vi "message.vi"(5 "visible?":bool=TRUE, 8 "error in (no error)":errorcluster, 9 "BG slider":u32(colorbox)=16711680, 10 "text":string, 11 "control references in":T1) -> (0 "error out":errorcluster, 2 "previous text":string, 3 "control references out":T1, 4 "previously visible?":bool=TRUE, 6 "previous BG colour":u32(colorbox)=16711680)   [LabVIEW 2010]
uses:
  type_definitions/clusters/controls_refs.ctl
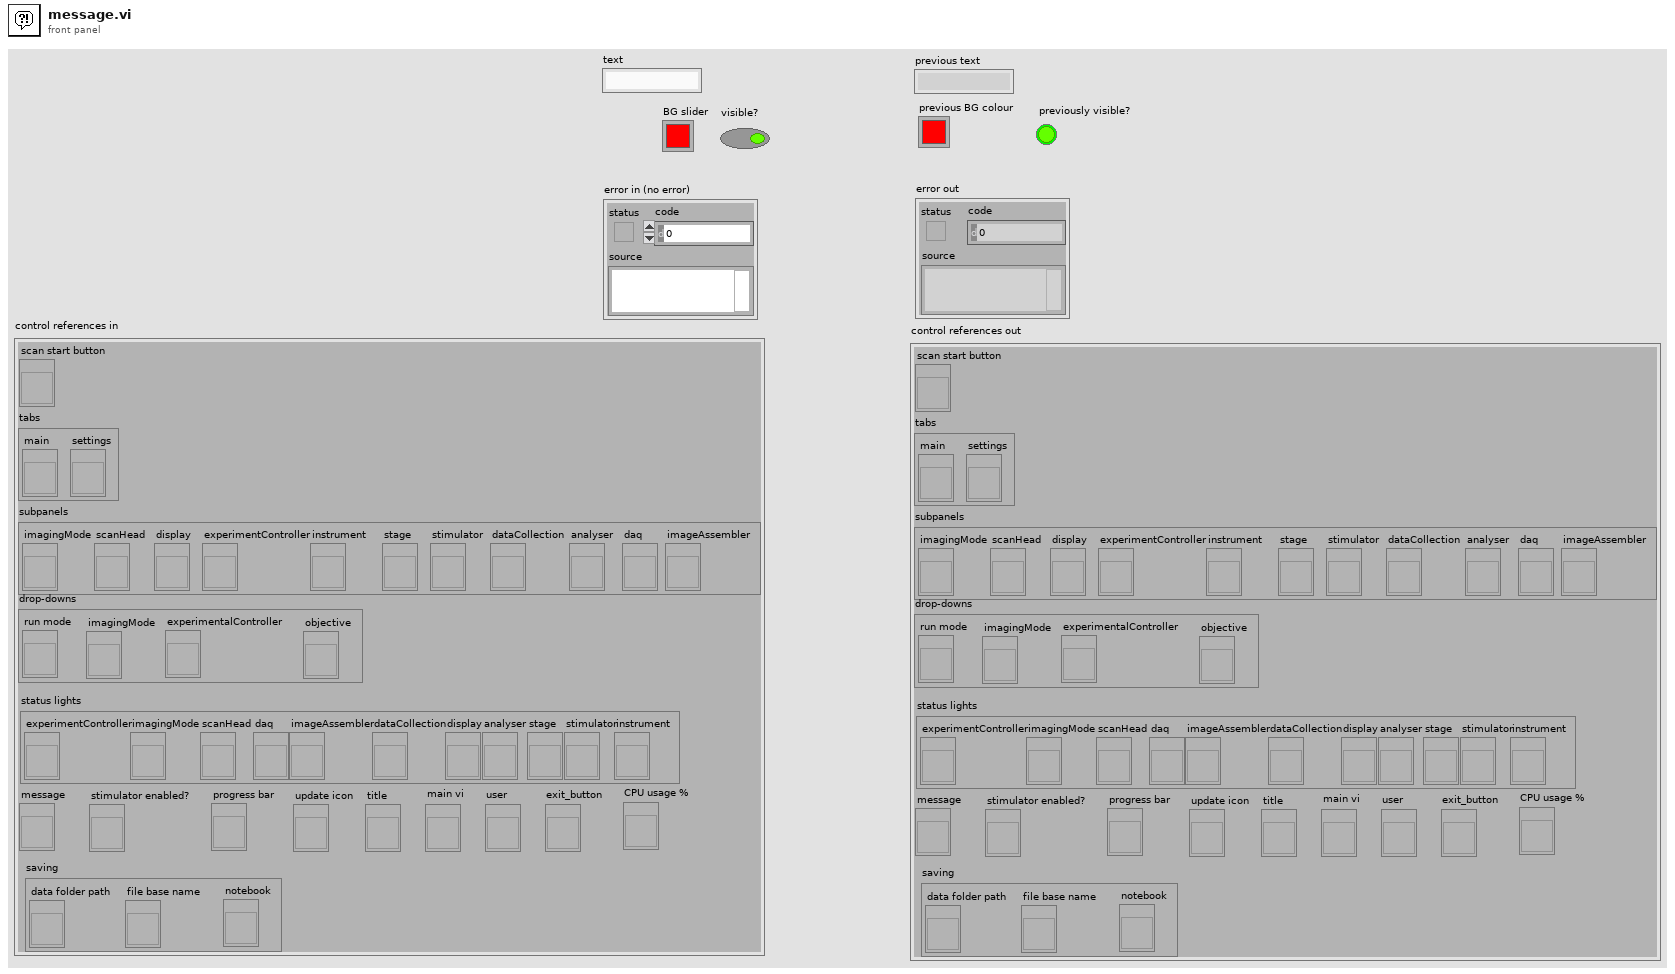
[diagram p1: front panel]
types:
  T1 = typedef "controls_refs.ctl" = cluster{"scan start button":refnum<vi>, "tabs":cluster{"main":refnum<vi>, "settings":refnum<vi>}, "subpanels":cluster{"imagingMode":refnum<vi>, "scanHead":refnum<vi>, "display":refnum<vi>, "experimentController":refnum<vi>, "instrument":refnum<vi>, "stage":refnum<vi>, "stimulator":refnum<vi>, "dataCollection":refnum<vi>, "analyser":refnum<vi>, "daq":refnum<vi>, "imageAssembler":refnum<vi>}, "drop-downs":cluster{"run mode":refnum<vi>, "imagingMode":refnum<vi>, "experimentalController":refnum<vi>, "objective":refnum<vi>}, "status lights":cluster{"experimentController":refnum<vi>, "imagingMode":refnum<vi>, "scanHead":refnum<vi>, "daq":refnum<vi>, "imageAssembler":refnum<vi>, "dataCollection":refnum<vi>, "display":refnum<vi>, "analyser":refnum<vi>, "stage":refnum<vi>, "stimulator":refnum<vi>, "instrument":refnum<vi>}, "message":refnum<vi>, "stimulator enabled?":refnum<vi>, "saving":cluster{"data folder path":refnum<vi>, "file base name":refnum<vi>, "notebook":refnum<vi>}, "progress bar":refnum<vi>, "update icon":refnum<vi>, "title":refnum<vi>, "main vi":refnum<vi>, "user":refnum<vi>, "exit_button":refnum<vi>, "CPU usage %":refnum<vi>}
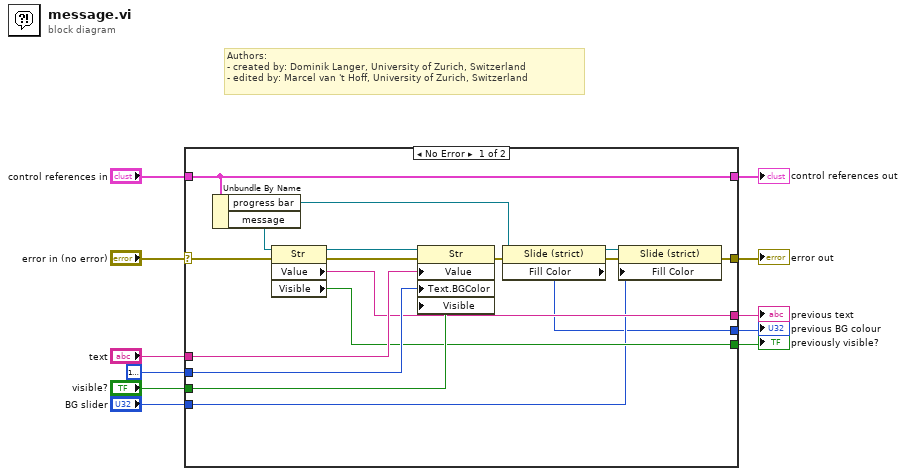
[diagram p0: block diagram]
diagram:
  # "Authors: \n- created by: Dominik Langer, University of Zurich, Switzerland\n- edited by: Marcel van 't Hoff, University of Zurich, Switzerland"
  n1 = case shown="No Error" "error in (no error)" {
    selector: "error in (no error)" -> [w21 w30]
    tunnel: [w18 w30] -> w10
    tunnel: "text" -> [w28 _]
    tunnel: u32 16777216 ("BG colour") -> [w27 _]
    tunnel: "visible?" -> [w26 _]
    tunnel: [w23 _] -> w5
    tunnel: [w12 _] -> w6
    tunnel: [w22 _] -> w4
    tunnel: "control references in" -> [w19 w29]
    tunnel: [w19 w29] -> w1
    tunnel: "BG slider" -> [w17 _]
    frame No Error {
      n2 = Unbundle By Name(w19) -> ("progress bar"=w14:refnum<vi>, "message"=w20:refnum<vi>)
      n3 = property class="Str"(reference=w20, error in=w21) -> (reference out=w24:refnum<vi>, error out=w25:errorcluster, "Value"=w23:string, "Visible"=w22:bool)
      n4 = property class="Str"(reference=w24, error in=w25, "Value"=w28, "Text.BGColor"=w27, "Visible"=w26) -> (error out=w16:errorcluster)  [unwired: 1 out]
      n5 = property class="Slide (strict)"(reference=w14, error in=w16) -> (reference out=w13:refnum<vi>, error out=w15:errorcluster, "Fill Color"=w12:u32)
      n6 = property class="Slide (strict)"(reference=w13, error in=w15, "Fill Color"=w17) -> (error out=w18:errorcluster)  [unwired: 1 out]
    }
    frame Error {
    }
  }
  "error out" <- w10
  "previous text" <- w5
  "previous BG colour" <- w6
  "previously visible?" <- w4
  "control references out" <- w1
